vi "Set LED Indicator.vi"(0 "LED On":bool) -> ()   [LabVIEW 2013]
doc: "Set the color of the indicator LED strip to our alliance color and enable it if the given condition is true. This condition will change during the match to indicate certain conditions."
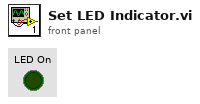
[diagram p1: front panel]
types:
  T1 = typedef "WPI_DriverStationAllianceInfo.ctl" = enum16{"Red", "Blue", "Invalid"}
  T2 = typedef "WPI_DigitalOutputDevRef.ctl" = cluster{"Digital Module":T3, "DIO Channel":T4, "DevStatus":errorcluster}
  T3 = typedef "FPGA_TypedefDigitalModule.ctl" = enum16{"Digital Module 1", "Digital Module 2"}
  T4 = typedef "FPGA_DIOChannel.ctl" = enum8{"DIO 1", "DIO 2", "DIO 3", "DIO 4", "DIO 5", "DIO 6", "DIO 7", "DIO 8", "DIO 9", "DIO 10", "DIO 11", "DIO 12", "DIO 13", "DIO 14", "Invalid"}
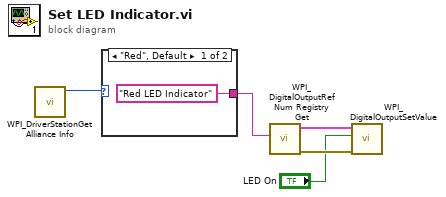
[diagram p0: block diagram]
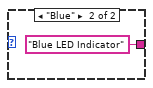
[diagram p2: hidden frame]
diagram:
  n1 = call <vilib>:"WPI_DriverStationGet Alliance Info.vi"() -> ("Alliance"=w4:T1)  [unwired: 10 in, 1 out]
  n2 = case shown="\"Red\", Default" w4 {
    tunnel: ["Red LED Indicator" ("refnum name") "Blue LED Indicator" ("refnum name")] -> w3
    frame "Red", Default {
    }
    frame "Blue" {
    }
  }
  n3 = call <vilib>:"WPI_DigitalOutputRefNum Registry Get.vi"("refnum name"=w3) -> ("error out"=w5:errorcluster, "DigitalOutputDevRef"=w1:T2)  [unwired: 9 in]
  n4 = call <vilib>:"WPI_DigitalOutputSetValue.vi"("error in (no error)"=w5, "Value"="LED On", "DigitalOutputDevRef"=w1) -> ()  [unwired: 7 in, 2 out]
